vi "TrajectoryIssueCmd.vi"(11 "Command":string) -> ()   [LabVIEW 2023]
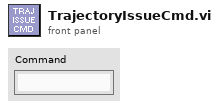
[diagram p1: front panel]
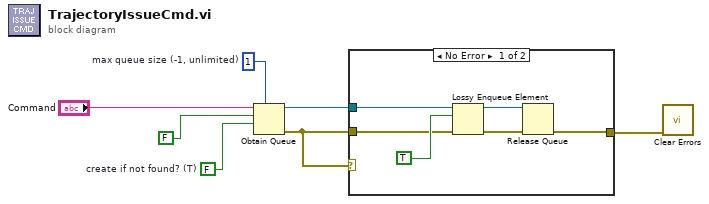
[diagram p0: block diagram]
diagram:
  w6 = FALSE  # create if not found? (T)
  w5 = 1  # max queue size (-1, unlimited)
  n1 = Obtain Queue(max queue size (-1, unlimited)=w5, name (unnamed)="Command", element data type=FALSE, create if not found? (T)=w6) -> (queue out=w3:refnum<queue>, error out=w1:errorcluster)  [unwired: 1 in, 1 out]
  n2 = case shown="No Error" w1 {
    tunnel: w3 -> [w11 _]
    tunnel: [w9 w14] -> w2
    tunnel: w1 -> [w8 w14]
    frame No Error {
      n3 = Lossy Enqueue Element(queue=w11, element=TRUE, error in (no error)=w8) -> (queue out=w13:refnum<queue>, error out=w12:errorcluster)  [unwired: 2 out]
      n4 = Release Queue(queue=w13, error in (no error)=w12) -> (error out=w9:errorcluster)  [unwired: 1 in, 2 out]
    }
    frame Error {
    }
  }
  n5 = call <vilib>:"Clear Errors.vi"("error in (no error)"=w2) -> ()  [unwired: 5 in, 2 out]
